vi "Robot Global Data.vi"() -> ()   [LabVIEW 2013]
doc: "This global VI can contain as many global variables as you need. Place a control on the panel, give it a good name. To read or write to it from a VI, drag the icon to the diagram of that VI. You can also drag from the project. Click on the node to change which global you access. You shouldn't have multiple locations writing to a global or it will cause a race-condition."
uses:
  <vilib>/Rock Robotics/WPI/Camera/WPI_CameraImageSize.ctl
  <vilib>/Rock Robotics/WPI/DriverStation/WPI_DriverStationRobotMode2.ctl
panel:
  in  "NumAutoRuns":u32
  in  "cAutoDistance":bool
  in  "cAutoRotate":bool
  in  "UseQueue?":bool
  in  "ImagesProcessed":dbl
  in  "ImagesHot":dbl
  in  "Andrew":bool
  in  "Andrew2":bool
  in  "Andrew1":bool
  in  "cStraightDrive":bool
  in  "TankDriveRight":dbl=-0.007874015748031496
  in  "TankDriveLeft":dbl=0.023622047244094488
  in  "cHalfDrive":bool
  in  "cSonicShifter":bool
  in  "cFireLauncher":bool
  in  "cClimbWeight":bool
  in  "Robot Mode":T1=enum."Timeout"
  in  "LED toggle rate (ms)":u32=500
  in  "image size":T2=enum."320x240"
  in  "Enable Vision":bool
  # "DRIVE"
  # "CLIMB"
  # "SHOOTER"
  # "AUTOALIGN"
  # "4"
  # "3"
  # "2"
  # "1"
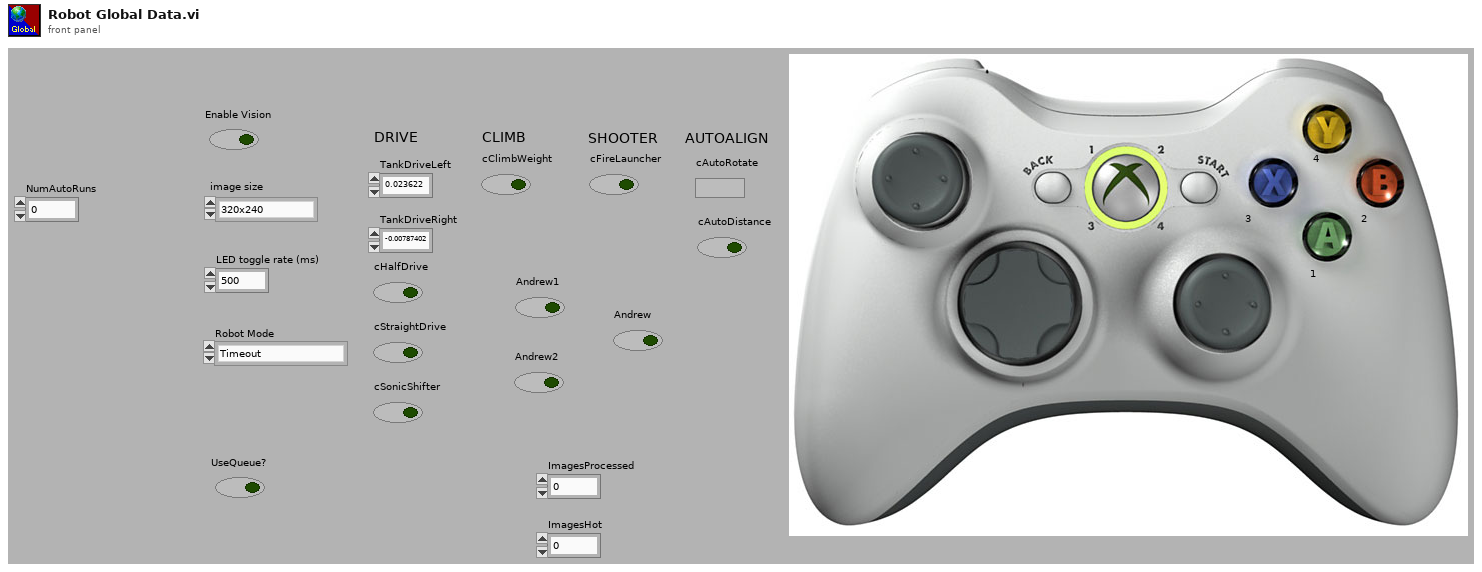
[diagram p1: front panel]
types:
  T1 = typedef "WPI_DriverStationRobotMode2.ctl" = enum16{"Autonomous Disabled", "Autonomous Enabled", "Teleop Disabled", "Teleop Enabled", "Timeout", "Finish", "Test Disabled", "Test Enabled"}
  T2 = typedef "WPI_CameraImageSize.ctl" = enum16{"640x480", "320x240", "160x120"}
diagram:
